vi "configure.vi"(8 "error in (no error)":errorcluster, 11 "LightSourceMG090910LightEmittingDiode in":refnum<class "LightSourceMG090910LightEmittingDiode.lvclass">) -> (0 "error out":errorcluster, 3 "LightSourceMG090910LightEmittingDiode out":refnum<class "LightSourceMG090910LightEmittingDiode.lvclass">)   [LabVIEW 2010, in "LightSourceMG090910LightEmittingDiode.lvclass"]
doc: "The dynamic dispatch version of this VI loads and displays the configuration file associated with the plug-in object. The user modify and save the configuration data."
uses:
  LightSourceMG090910LightEmittingDiode.lvclass
  LightSourceMG090910LightEmittingDiode.lvclass/LightSourceMG090910LightEmittingDiode.ctl
  common/classes/GenericComponent/GenericComponent/GenericComponent.lvclass
panel:
  out "LSID":string
  out "Configuration":string
  in  "cancel button":bool
  in  "save button":bool
  in  "Serial number":string
  in  "Model":string
  in  "Manufacturer":string
  # "Configure LightSourceMG090910LightEmittingDiode"
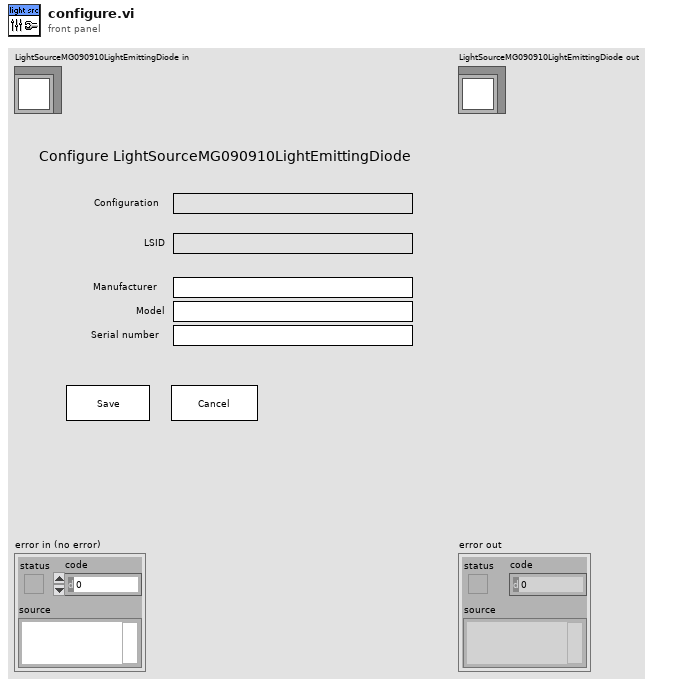
[diagram p1: front panel]
types:
  T1 = typedef "LSID_cluster.ctl" = cluster{"identifier":string, "revision":i32}
  T2 = typedef "LightSourceMG090910LightEmittingDiode.lvclass/config_data_cluster.ctl" = cluster{"LSID":T1, "manufacturer specification":T3}
  T3 = typedef "GenericComponent.lvclass/manufacturer_specification_cluster.ctl" = cluster{"manufacturer":string, "model":string, "serial number":string, "lot number":string}
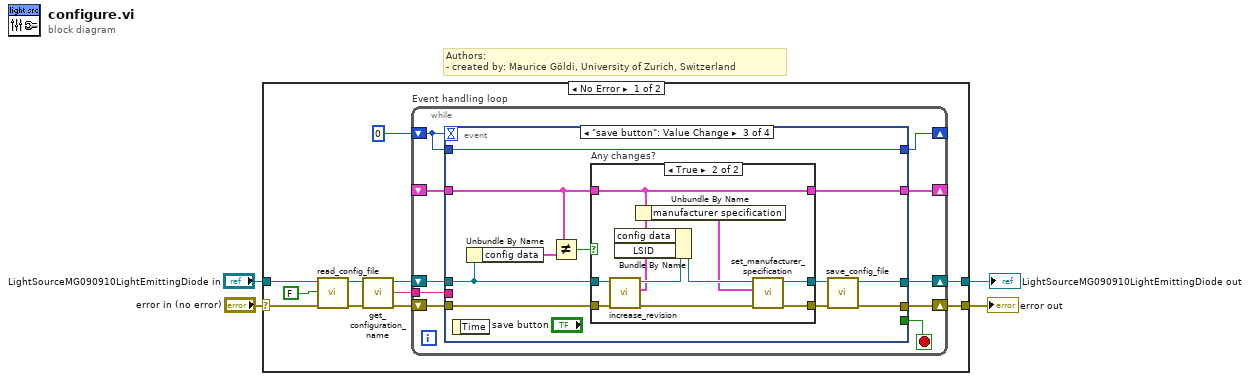
[diagram p0: block diagram]
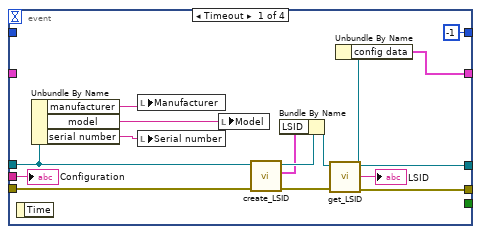
[diagram p2: hidden frame]
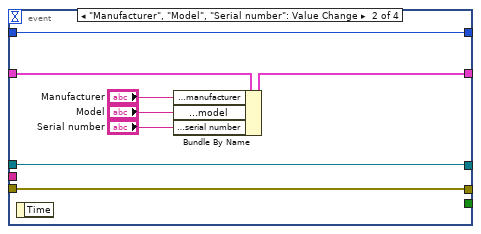
[diagram p3: hidden frame]
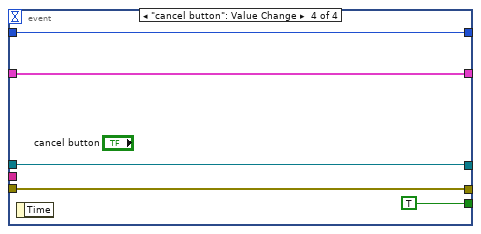
[diagram p5: hidden frame]
diagram:
  # "Authors: \n- created by: Maurice Göldi, University of Zurich, Switzerland"
  n1 = case shown="No Error" "error in (no error)" {
    selector: "error in (no error)" -> [w10 w79]
    tunnel: [w15 w79] -> w4
    tunnel: [w14 w78] -> w3
    tunnel: "LightSourceMG090910LightEmittingDiode in" -> [w9 w78]
    frame No Error {
      n2 = call-dynamic "read_config_file.vi"("error in (no error)"=w10, "force load?"=FALSE, "GenericPlugin in"=w9) -> ("error out"=w13:errorcluster, "GenericPlugin out"=w12:refnum<class "LightSourceMG090910LightEmittingDiode.lvclass">)  [unwired: 7 in]
      n3 = call "get_configuration_name.vi"("error in (no error)"=w13, "GenericPlugin.lvclass in"=w12) -> ("error out"=w7:errorcluster, "configuration name"=w6:string, "GenericPlugin.lvclass out"=w8:refnum<class "LightSourceMG090910LightEmittingDiode.lvclass">)  [unwired: 7 in]
      n4 = while "Event handling loop" {
        shift-right: [w24] -> w14
        shift-left: w8 -> [w23]
        shift-right: [w25] -> w15
        shift-left: w7 -> [w22]
        tunnel: w6 -> [w21]
        shift-right: [w20] -> _
        shift-left: _ -> [w19]
        shift-right: [w17] -> _
        shift-left: 0 -> [w18]
        stop <- w16 stop-if-true
        n5 = event shown="[2] \"save button\": Value Change" {
          selector: _ -> [_ _ _ _]
          dyn-events: _ -> [_ _ _ _]
          timeout: w18 -> [_ _ _ _]
          tunnel: [w31 w48 w53 w74] -> w25
          tunnel: [w28 w43 w51 w75] -> w24
          tunnel: w23 -> [w30 w43 w56 w75]
          tunnel: w22 -> [w32 w48 w57 w74]
          tunnel: w21 -> [w40 _ _ _]
          tunnel: [w27 w41 w49 w77] -> w20
          tunnel: w19 -> [_ w42 w50 w77]
          tunnel: w18 -> [_ w47 w59 w76]
          tunnel: [-1 w47 w59 w76] -> w17
          tunnel: [_ _ _ TRUE] -> w16
          event Timeout {
            n6 = event-data() -> ()  [unwired: 1 in, 1 out]
            n7 = Unbundle By Name(w30) -> ("manufacturer"=w39:string, "model"=w38:string, "serial number"=w37:string)
            n8 = local write "Manufacturer"(w39) -> ()
            n9 = local write "Serial number"(w37) -> ()
            n10 = local write "Model"(w38) -> ()
            n11 = call-dynamic "create_LSID.vi"("error in (no error)"=w32, "GenericPlugin in"=w30) -> ("error out"=w36:errorcluster, "current LSID"=w33:T1, "GenericPlugin out"=w35:refnum<class "LightSourceMG090910LightEmittingDiode.lvclass">)  [unwired: 7 in]
            n12 = Bundle By Name(cluster=w35, "LSID"=w33) -> (w34:refnum<class "LightSourceMG090910LightEmittingDiode.lvclass">)
            n13 = call-dynamic "get_LSID.vi"("error in (no error)"=w36, "GenericPlugin in"=w34) -> ("error out"=w31:errorcluster, "LSID (string)"=→"LSID":string, "GenericPlugin out"=w28:refnum<class "LightSourceMG090910LightEmittingDiode.lvclass">)  [unwired: 6 in, 1 out]
            n14 = Unbundle By Name(w28) -> ("config data"=w27:T2)
            "Configuration" <- w40
          }
          event "Manufacturer", "Model", "Serial number": Value Change {
            n15 = event-data() -> ()  [unwired: 1 in, 1 out]
            n16 = Bundle By Name(cluster=w42, "manufacturer specification.manufacturer"="Manufacturer", "manufacturer specification.model"="Model", "manufacturer specification.serial number"="Serial number") -> (w41:T2)
          }
          event "save button": Value Change {
            n17 = event-data() -> ()  [unwired: 1 in, 1 out]
            n18 = Unbundle By Name(w56) -> ("config data"=w58:T2)
            n19 = Not Equal?(x=w50, y=w58) -> (x != y?=w55:bool)
            n20 = case "Any changes?" shown="True" w55 {
              tunnel: w57 -> [w62 w72]
              tunnel: [w62 w67] -> w54
              tunnel: w56 -> [w61 w71]
              tunnel: [w61 w65] -> w52
              tunnel: w50 -> [w60 w63]
              tunnel: [w60 w63] -> w49
              frame False {
              }
              frame True {
                n21 = call-dynamic "increase_revision.vi"("error in (no error)"=w72, "GenericPlugin in"=w71) -> ("error out"=w68:errorcluster, "new LSID"=w69:T1, "GenericPlugin out"=w70:refnum<class "LightSourceMG090910LightEmittingDiode.lvclass">)  [unwired: 7 in]
                n22 = Bundle By Name(cluster=w70, "config data"=w63, "LSID"=w69) -> (w66:refnum<class "LightSourceMG090910LightEmittingDiode.lvclass">)
                n23 = Unbundle By Name(w63) -> ("manufacturer specification"=w64:T3)
                n24 = call-dynamic "set_manufacturer_specification.vi"("error in (no error)"=w68, "manufacturer specification"=w64, "GenericPlugin in"=w66) -> ("error out"=w67:errorcluster, "GenericPlugin out"=w65:refnum<class "LightSourceMG090910LightEmittingDiode.lvclass">)  [unwired: 7 in]
              }
            }
            n25 = call-dynamic "save_config_file.vi"("error in (no error)"=w54, "GenericPlugin in"=w52) -> ("error out"=w53:errorcluster, "GenericPlugin out"=w51:refnum<class "LightSourceMG090910LightEmittingDiode.lvclass">)  [unwired: 8 in]
          }
          event "cancel button": Value Change {
            n26 = event-data() -> ()  [unwired: 1 in, 1 out]
          }
        }
      }
    }
    frame Error {
    }
  }
  "error out" <- w4
  "LightSourceMG090910LightEmittingDiode out" <- w3
